vi "Error Tree Value Change.vi"(8 "error in (no error)":errorcluster, 10 "Error Tree":string, 11 "Error Log in":refnum<class "Error Log.lvclass">) -> (0 "error out":errorcluster, 3 "Error Log out":refnum<class "Error Log.lvclass">)   [LabVIEW 2023, in "Data Analysis.lvlib" / "Error Log.lvlib" / "Error Log.lvclass"]
uses:
  Error Log.lvclass
  Error Log.lvclass/Error Log.ctl
  HardwareAbstractionLayer_LVOOP/Database/Database.lvclass
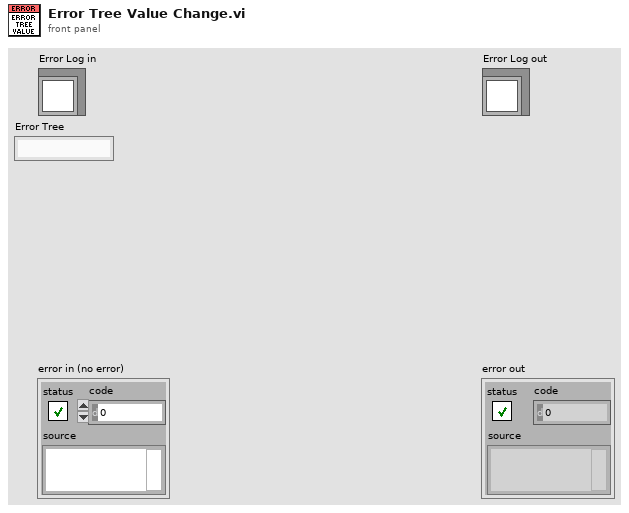
[diagram p1: front panel]
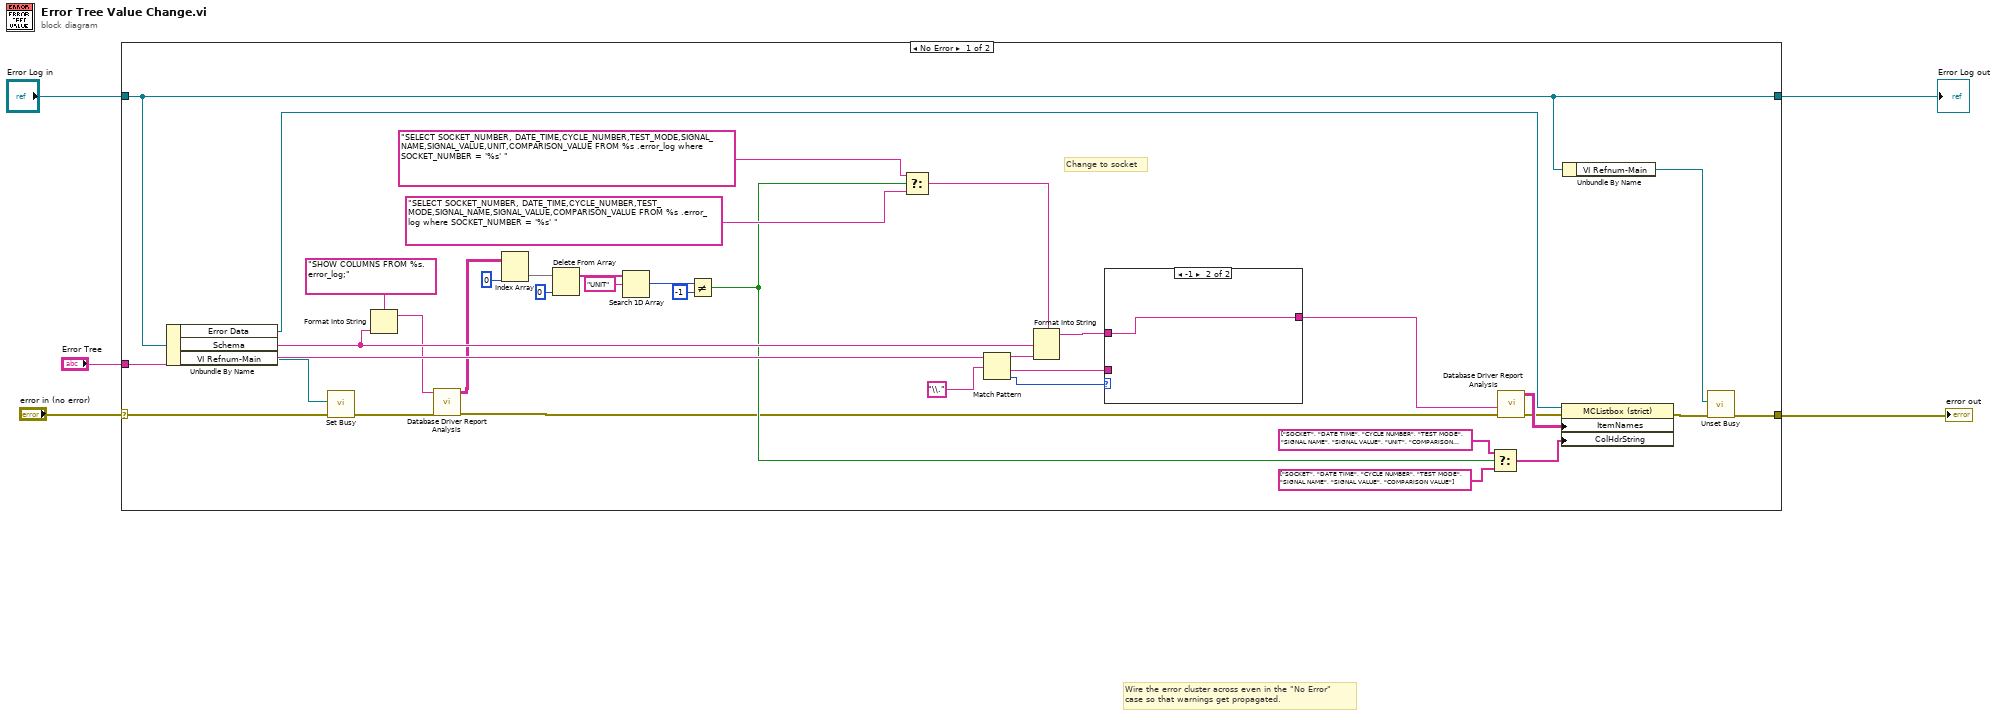
[diagram p0: block diagram]
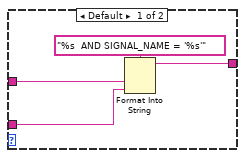
[diagram p2: hidden frame]
diagram:
  # "Wire the error cluster across even in the \"No Error\"\ncase so that warnings get propagated."
  n1 = case shown="No Error" "error in (no error)" {
    selector: "error in (no error)" -> [w30 w48]
    tunnel: [w26 w48] -> w4
    tunnel: [w29 w47] -> w2
    tunnel: "Error Log in" -> [w29 w47]
    tunnel: "Error Tree" -> [w32 _]
    frame No Error {
      # "Change to socket"
      n2 = Unbundle By Name(w29) -> ("Error Data"=w33:refnum<vi>, "Schema"=w21:string, "VI Refnum-Main"=w31:refnum<vi>)
      n3 = call <vilib>:"Set Busy.vi"("error in (no error)"=w30, "VI reference (current VI)"=w31) -> ("error out"=w9:errorcluster)  [unwired: 8 in, 1 out]
      n4 = Format Into String(format string="SHOW COLUMNS FROM %s.error_log;" ("SQL query"), w21) -> (resulting string=w7:string)  [unwired: 2 in, 1 out]
      n5 = call "Database Driver Report Analysis.vi"("error in"=w9, "table"=w7) -> ("error out"=w8:errorcluster, "data"=w6:string[][])  [unwired: 6 in, 2 out]
      n6 = Index Array(array=w6, index (col)=0 ("disabled index (col)")) -> (element=w25:string[])  [unwired: 1 in]
      n7 = Delete From Array(array=w25, index=0) -> (array with subset deleted=w20:string[])  [unwired: 1 in, 1 out]
      n8 = Search 1D Array(1D array=w20, element="UNIT") -> (index of element=w18:i32)  [unwired: 1 in]
      n9 = Not Equal?(x=w18, y=-1) -> (x != y?=w10:bool)
      n10 = Select(t="SELECT SOCKET_NUMBER, DATE_TIME,CYCLE_NUMBER,TEST_MODE,SIGNAL_NAME,SIGNAL_VALUE,UNIT,COMPARISON_VALUE FROM %s .error_log where SOCKET_NUMBER = '%s' " ("SQL query"), s=w10, f="SELECT SOCKET_NUMBER, DATE_TIME,CYCLE_NUMBER,TEST_MODE,SIGNAL_NAME,SIGNAL_VALUE,COMPARISON_VALUE FROM %s .error_log where SOCKET_NUMBER = '%s' " ("SQL query")) -> (s? t:f=w16:string)
      n11 = Match Pattern(string=w32, regular expression="\\.") -> (before substring=w40:string, after substring=w34:string, offset past match=w37:i32)  [unwired: 1 in, 1 out]
      n12 = Format Into String(format string=w16, w21, w40) -> (resulting string=w39:string)  [unwired: 2 in, 1 out]
      n13 = case shown="-1" w37 {
        tunnel: w39 -> [w44 w46]
        tunnel: [w42 w46] -> w38
        tunnel: w34 -> [w43 _]
        frame Default {
          n14 = Format Into String(format string="%s  AND SIGNAL_NAME = '%s'" ("SQL query"), w44, w43) -> (resulting string=w42:string)  [unwired: 2 in, 1 out]
        }
        frame -1 {
        }
      }
      n15 = Select(t=string[] ["SOCKET", "DATE TIME", "CYCLE NUMBER", "TEST MODE", "SIGNAL NAME", "SIGNAL VALUE", "UNIT", "COMPARISON VALUE"] ("Column Header Strings[]"), s=w10, f=string[] ["SOCKET", "DATE TIME", "CYCLE NUMBER", "TEST MODE", "SIGNAL NAME", "SIGNAL VALUE", "COMPARISON VALUE"] ("Column Header Strings[]")) -> (s? t:f=w11:string[])
      n16 = call "Database Driver Report Analysis.vi"("error in"=w8, "SQL query"=w38) -> ("error out"=w35:errorcluster, "data"=w36:string[][])  [unwired: 6 in, 2 out]
      n17 = property class="MCListbox (strict)"(reference=w33, error in=w35, "ItemNames"=w36, "ColHdrString"=w11) -> (error out=w27:errorcluster)  [unwired: 1 out]
      n18 = Unbundle By Name(w29) -> ("VI Refnum-Main"=w28:refnum<vi>)
      n19 = call <vilib>:"Unset Busy.vi"("error in (no error)"=w27, "VI reference (current VI)"=w28) -> ("error out"=w26:errorcluster)  [unwired: 9 in]
    }
    frame Error {
    }
  }
  "error out" <- w4
  "Error Log out" <- w2
